vi "Car Wash.vi"() -> ()   [LabVIEW 2015]
uses:
  Controls/Car Wash Indicators.ctl
  Controls/Wash Options.ctl
  Controls/All data cluster.ctl
  Controls/#status.ctl
  Car Wash (100929B-01)/USB Template (LV 8.6)/Car Wash/Controls/#timerstatus.ctl
panel:
  in  "Wash Options":T1
  out "error out":errorcluster
  in  "error in":errorcluster
  in  "Start":bool
  out "Elapsed Time":dbl format="%0.2f"
  in  "stop":bool
  out "Wash Entry":bool
  in  "Car Position Slider":u8(slide) max=3 scale=0.0..4.0
  out "Car Wash Indicators":T2
  # "Entry Console"
  # "Car Wash Display"
  # "Car Position Simulation"
  # "Pre-Soak\nH-P Wash\nL-P Wax\nSpot Free Rinse"
  # "Underbody Wash\nBug Remover"
  # "Tire Shine\nAir Dry"
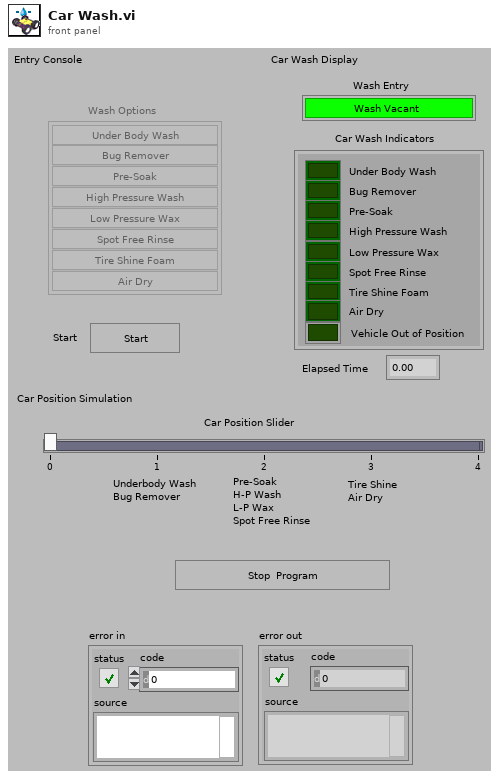
[diagram p1: front panel]
types:
  T1 = typedef "Wash Options.ctl" = cluster{"Underbody Wash":bool, "Bug Remover":bool, "Pre-Soak":bool, "High Pressure Wash":bool, "Low Pressure Wax":bool, "Spot Free Rinse":bool, "Tire Shine Foam":bool, "Air Dry":bool}
  T2 = typedef "Car Wash Indicators.ctl" = cluster{"Under Body Wash":bool, "Bug Remover":bool, "Pre-Soak":bool, "High Pressure Wash":bool, "Low Pressure Wax":bool, "Spot Free Rinse":bool, "Tire Shine Foam":bool, "Air Dry":bool, "Vehicle Out of Position":bool}
  T3 = typedef "#status.ctl" = enum16{"Error Under Range", "Skip", "Error", "Initialize", "End", "Air Dry", "Tire Shine Foam", "Spot Free Rinse", "Low Pressure Wax", "High Pressure Wash", "Pre-Soak", "Bug Remover", "Under Body Wash", "Start", "Idle", "Exit"}
  T4 = typedef "All data cluster.ctl" = cluster{"Car Wash Indicators":T2, "Wash Entry":bool, "Elapsed Time":dbl, "times":cluster{"UBW":dbl, "Bug Remover":dbl, "Pre-Soak":dbl, "HPW":dbl, "LPW":dbl, "TSF":dbl, "AD":dbl, "SFR":dbl}}
  T5 = cluster{"UBW":dbl, "Bug Remover":dbl, "Pre-Soak":dbl, "HPW":dbl, "LPW":dbl, "TSF":dbl, "AD":dbl, "SFR":dbl}
  T6 = enum8{"Enabled", "Disabled", "Disabled and Grayed Out"}
  T7 = typedef "#timerstatus.ctl" = enum16{"pause", "reset", "start"}
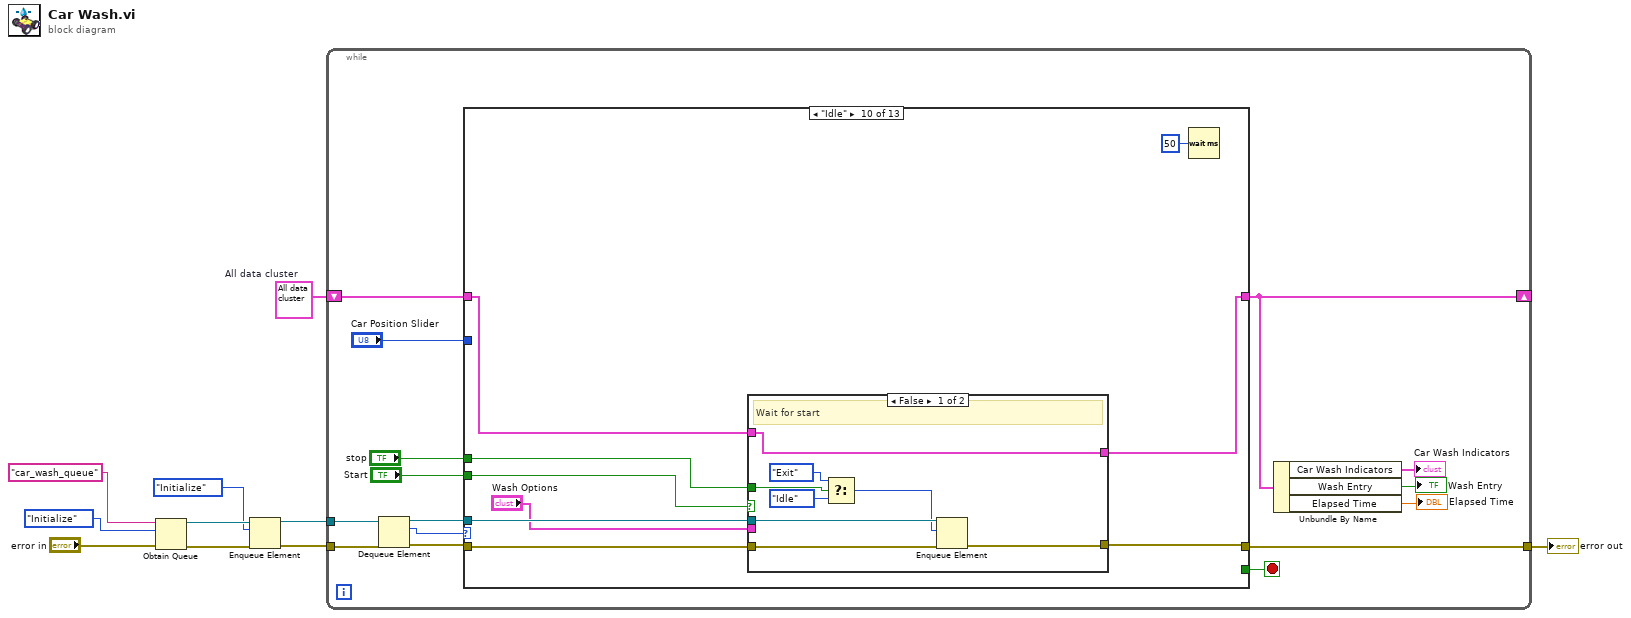
[diagram p0: block diagram]
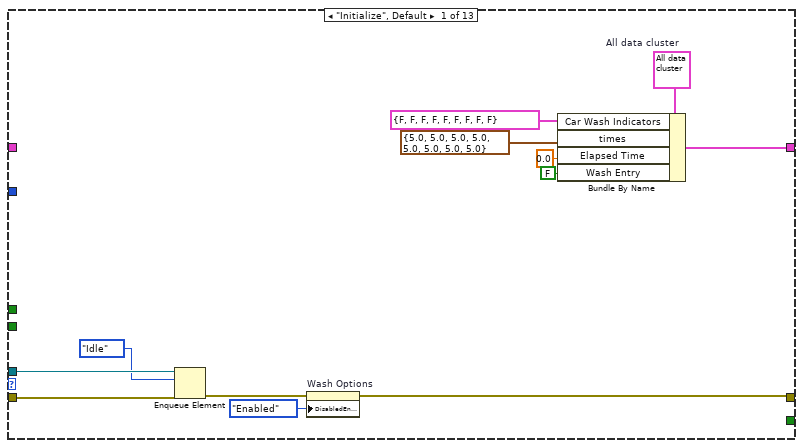
[diagram p2: hidden frame]
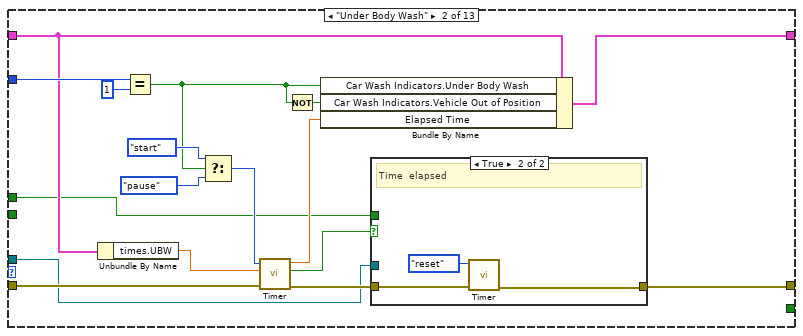
[diagram p3: hidden frame]
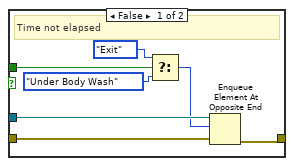
[diagram p4: hidden frame]
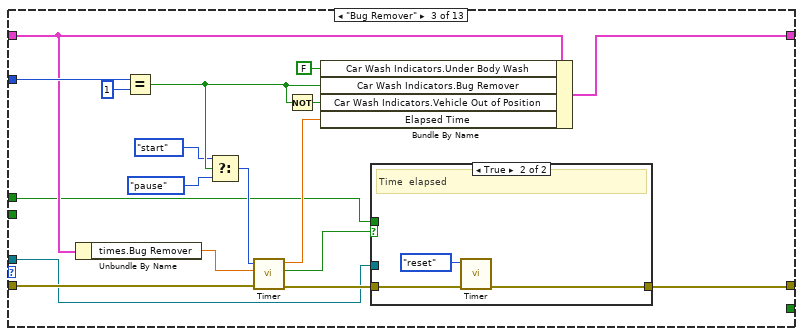
[diagram p5: hidden frame]
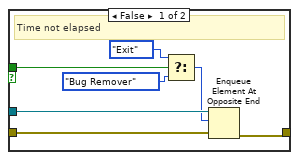
[diagram p6: hidden frame]
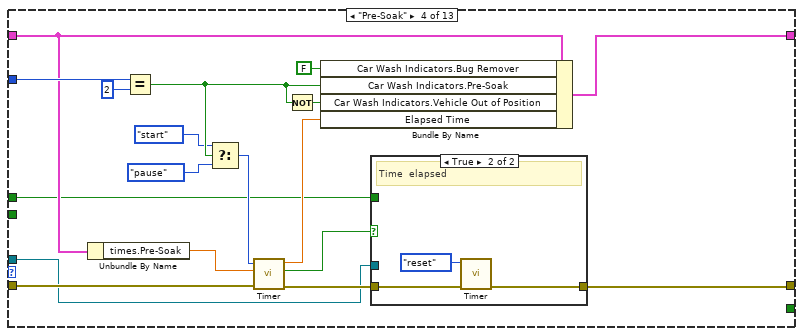
[diagram p7: hidden frame]
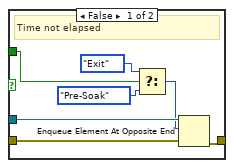
[diagram p8: hidden frame]
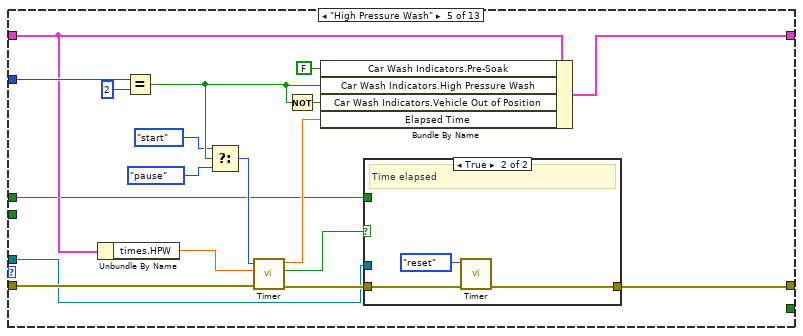
[diagram p9: hidden frame]
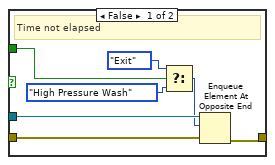
[diagram p10: hidden frame]
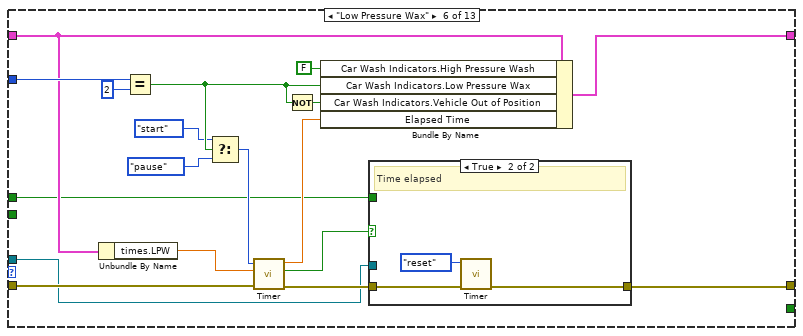
[diagram p11: hidden frame]
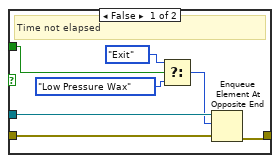
[diagram p12: hidden frame]
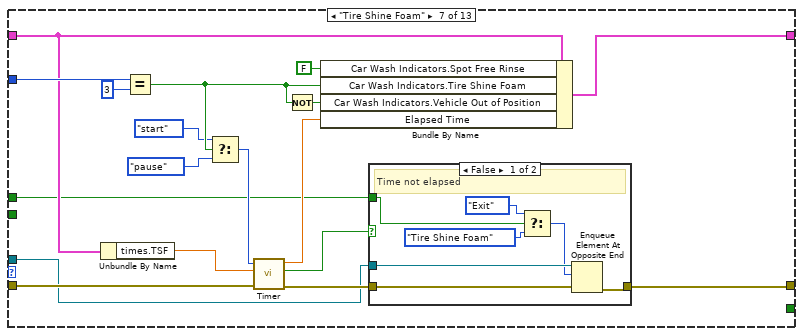
[diagram p13: hidden frame]
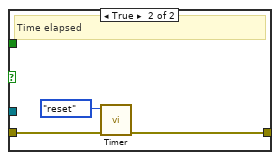
[diagram p14: hidden frame]
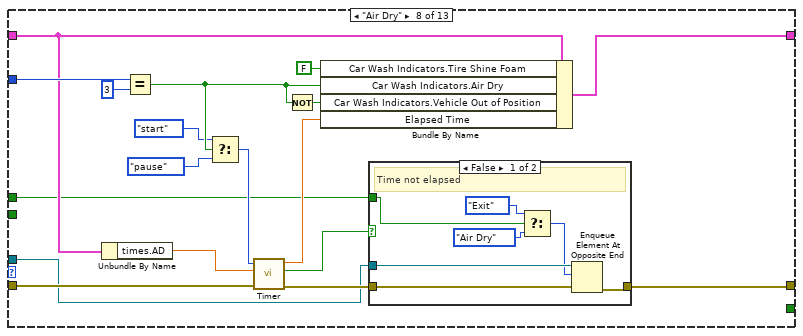
[diagram p15: hidden frame]
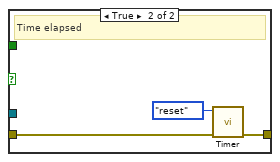
[diagram p16: hidden frame]
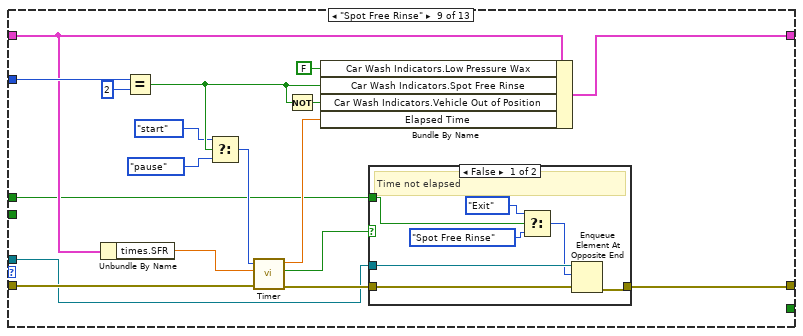
[diagram p17: hidden frame]
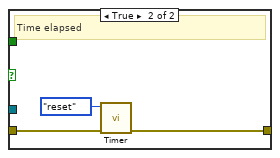
[diagram p18: hidden frame]
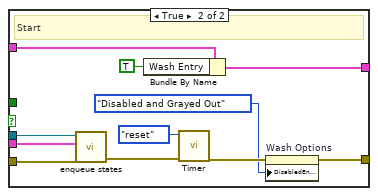
[diagram p19: hidden frame]
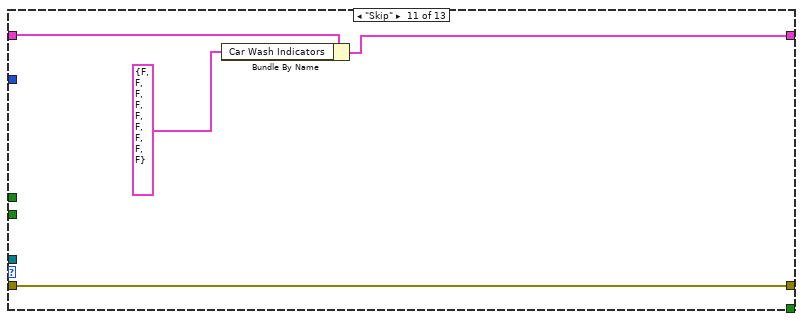
[diagram p20: hidden frame]
diagram:
  w10 = T4 {"Car Wash Indicators"={"Under Body Wash"=FALSE, "Bug Remover"=FALSE, "Pre-Soak"=FALSE, "High Pressure Wash"=FALSE, "Low Pressure Wax"=FALSE, "Spot Free Rinse"=FALSE, "Tire Shine Foam"=FALSE, "Air Dry"=FALSE, "Vehicle Out of Position"=FALSE}, "Wash Entry"=FALSE, "Elapsed Time"=0.0, "times"={"UBW"=0.0, "Bug Remover"=0.0, "Pre-Soak"=0.0, "HPW"=0.0, "LPW"=0.0, "TSF"=0.0, "AD"=0.0, "SFR"=0.0}}  # All data cluster
  n1 = Obtain Queue(name (unnamed)="car_wash_queue", element data type=#status."Initialize" ("status"), error in (no error)="error in") -> (queue out=w3:refnum<queue>, error out=w5:errorcluster)  [unwired: 2 in, 1 out]
  n2 = Enqueue Element(queue=w3, element=#status."Initialize" ("status"), error in (no error)=w5) -> (queue out=w1:refnum<queue>, error out=w4:errorcluster)  [unwired: 1 in, 1 out]
  n3 = while {
    shift-right: [w23] -> _
    shift-left: w10 -> [w24]
    tunnel: w4 -> [w18]
    tunnel: [w19] -> w9
    tunnel: w1 -> [w16]
    stop <- w25 stop-if-true
    n4 = Dequeue Element(queue=w16, error in (no error)=w18) -> (queue out=w15:refnum<queue>, element=w14:T3, error out=w17:errorcluster)  [unwired: 1 in, 1 out]
    n5 = case shown="\"Idle\"" w14 {
      tunnel: [_ _ _ _ _ _ _ _ _ _ _ _ TRUE] -> w25
      tunnel: w24 -> [_ w50 w78 w106 w134 w162 w190 w218 w246 w262 w291 w298 w317]
      tunnel: [w33 w47 w75 w103 w131 w159 w187 w215 w243 w261 w289 w295 w317] -> w23
      tunnel: w17 -> [w32 w54 w82 w110 w138 w166 w194 w222 w250 w269 w292 w304 w318]
      tunnel: [w28 w45 w73 w101 w129 w157 w185 w213 w241 w267 w292 w302 w318] -> w19
      tunnel: w15 -> [w31 w43 w71 w99 w127 w155 w183 w211 w239 w268 _ w303 _]
      tunnel: "Start" -> [_ _ _ _ _ _ _ _ _ w266 _ _ _]
      tunnel: "stop" -> [_ w38 w65 w93 w121 w149 w177 w205 w233 w265 _ _ _]
      tunnel: "Car Position Slider" -> [_ w52 w80 w108 w136 w164 w192 w220 w248 _ _ w300 _]
      frame "Initialize", Default {
        w37 = T4 {"Car Wash Indicators"={"Under Body Wash"=FALSE, "Bug Remover"=FALSE, "Pre-Soak"=FALSE, "High Pressure Wash"=FALSE, "Low Pressure Wax"=FALSE, "Spot Free Rinse"=FALSE, "Tire Shine Foam"=FALSE, "Air Dry"=FALSE, "Vehicle Out of Position"=FALSE}, "Wash Entry"=TRUE, "Elapsed Time"=0.0, "times"={"UBW"=0.0, "Bug Remover"=0.0, "Pre-Soak"=0.0, "HPW"=0.0, "LPW"=0.0, "TSF"=0.0, "AD"=0.0, "SFR"=0.0}}  # All data cluster
        n6 = Enqueue Element(queue=w31, element=#status."Idle" ("status"), error in (no error)=w32) -> (error out=w29:errorcluster)  [unwired: 1 in, 2 out]
        n7 = property on="Wash Options" class="Clust (strict)"(error in=w29, "DisabledEnum"=T6."Enabled" ("Disabled")) -> (error out=w28:errorcluster)  [unwired: 1 in, 1 out]
        n8 = Bundle By Name(cluster=w37, "Car Wash Indicators"=T2 {"Under Body Wash"=FALSE, "Bug Remover"=FALSE, "Pre-Soak"=FALSE, "High Pressure Wash"=FALSE, "Low Pressure Wax"=FALSE, "Spot Free Rinse"=FALSE, "Tire Shine Foam"=FALSE, "Air Dry"=FALSE, "Vehicle Out of Position"=FALSE}, "times"=T5 {"UBW"=5.0, "Bug Remover"=5.0, "Pre-Soak"=5.0, "HPW"=5.0, "LPW"=5.0, "TSF"=5.0, "AD"=5.0, "SFR"=5.0}, "Elapsed Time"=0.0, "Wash Entry"=FALSE) -> (w33:T4)
      }
      frame "Under Body Wash" {
        n9 = Unbundle By Name(w50) -> ("times.UBW"=w53:dbl)
        n10 = Equal?(x=w52, y=u8 1) -> (x = y?=w40:bool)
        n11 = Select(t=#timerstatus."start" ("status"), s=w40, f=#timerstatus."pause" ("status")) -> (s? t:f=w39:T7)
        n12 = call "Timer.vi"("error in"=w54, "Time limit"=w53, "status"=w39) -> ("error out"=w46:errorcluster, "elapsed"=w44:bool, "elapsed time"=w49:dbl)  [unwired: 6 in]
        n13 = Not(x=w40) -> (.not. x?=w48:bool)
        n14 = Bundle By Name(cluster=w50, "Car Wash Indicators.Under Body Wash"=w40, "Car Wash Indicators.Vehicle Out of Position"=w48, "Elapsed Time"=w49) -> (w47:T4)
        n15 = case shown="True" w44 {
          tunnel: w46 -> [w61 w64]
          tunnel: [w60 w63] -> w45
          tunnel: w43 -> [w59 _]
          tunnel: w38 -> [w56 _]
          frame False {
            # "Time not elapsed"
            n16 = Select(t=#status."Exit" ("status"), s=w56, f=#status."Under Body Wash" ("element")) -> (s? t:f=w55:T3)
            n17 = Enqueue Element At Opposite End(queue=w59, element=w55, error in (no error)=w61) -> (error out=w60:errorcluster)  [unwired: 1 in, 2 out]
          }
          frame True {
            # "Time  elapsed"
            n18 = call "Timer.vi"("error in"=w64, "status"=#timerstatus."reset") -> ("error out"=w63:errorcluster)  [unwired: 7 in, 2 out]
          }
        }
      }
      frame "Bug Remover" {
        n19 = Unbundle By Name(w78) -> ("times.Bug Remover"=w81:dbl)
        n20 = Equal?(x=w80, y=u8 1) -> (x = y?=w69:bool)
        n21 = Select(t=#timerstatus."start" ("status"), s=w69, f=#timerstatus."pause" ("status")) -> (s? t:f=w66:T7)
        n22 = call "Timer.vi"("error in"=w82, "Time limit"=w81, "status"=w66) -> ("error out"=w74:errorcluster, "elapsed"=w72:bool, "elapsed time"=w77:dbl)  [unwired: 6 in]
        n23 = Not(x=w69) -> (.not. x?=w76:bool)
        n24 = Bundle By Name(cluster=w78, "Car Wash Indicators.Under Body Wash"=FALSE, "Car Wash Indicators.Bug Remover"=w69, "Car Wash Indicators.Vehicle Out of Position"=w76, "Elapsed Time"=w77) -> (w75:T4)
        n25 = case shown="True" w72 {
          tunnel: w74 -> [w89 w92]
          tunnel: [w88 w91] -> w73
          tunnel: w71 -> [w87 _]
          tunnel: w65 -> [w83 _]
          frame False {
            # "Time not elapsed"
            n26 = Select(t=#status."Exit" ("status"), s=w83, f=#status."Bug Remover" ("element")) -> (s? t:f=w84:T3)
            n27 = Enqueue Element At Opposite End(queue=w87, element=w84, error in (no error)=w89) -> (error out=w88:errorcluster)  [unwired: 1 in, 2 out]
          }
          frame True {
            # "Time  elapsed"
            n28 = call "Timer.vi"("error in"=w92, "status"=#timerstatus."reset") -> ("error out"=w91:errorcluster)  [unwired: 7 in, 2 out]
          }
        }
      }
      frame "Pre-Soak" {
        n29 = Unbundle By Name(w106) -> ("times.Pre-Soak"=w109:dbl)
        n30 = Equal?(x=w108, y=u8 2) -> (x = y?=w97:bool)
        n31 = Select(t=#timerstatus."start" ("status"), s=w97, f=#timerstatus."pause" ("status")) -> (s? t:f=w94:T7)
        n32 = call "Timer.vi"("error in"=w110, "Time limit"=w109, "status"=w94) -> ("error out"=w102:errorcluster, "elapsed"=w100:bool, "elapsed time"=w105:dbl)  [unwired: 6 in]
        n33 = Not(x=w97) -> (.not. x?=w104:bool)
        n34 = Bundle By Name(cluster=w106, "Car Wash Indicators.Bug Remover"=FALSE ("Car Wash Indicators.Under Body Wash"), "Car Wash Indicators.Pre-Soak"=w97, "Car Wash Indicators.Vehicle Out of Position"=w104, "Elapsed Time"=w105) -> (w103:T4)
        n35 = case shown="True" w100 {
          tunnel: w102 -> [w117 w120]
          tunnel: [w116 w119] -> w101
          tunnel: w99 -> [w115 _]
          tunnel: w93 -> [w111 _]
          frame False {
            # "Time not elapsed"
            n36 = Select(t=#status."Exit" ("status"), s=w111, f=#status."Pre-Soak" ("element")) -> (s? t:f=w112:T3)
            n37 = Enqueue Element At Opposite End(queue=w115, element=w112, error in (no error)=w117) -> (error out=w116:errorcluster)  [unwired: 1 in, 2 out]
          }
          frame True {
            # "Time  elapsed"
            n38 = call "Timer.vi"("error in"=w120, "status"=#timerstatus."reset") -> ("error out"=w119:errorcluster)  [unwired: 7 in, 2 out]
          }
        }
      }
      frame "High Pressure Wash" {
        n39 = Unbundle By Name(w134) -> ("times.HPW"=w137:dbl)
        n40 = Equal?(x=w136, y=u8 2) -> (x = y?=w125:bool)
        n41 = Select(t=#timerstatus."start" ("status"), s=w125, f=#timerstatus."pause" ("status")) -> (s? t:f=w122:T7)
        n42 = call "Timer.vi"("error in"=w138, "Time limit"=w137, "status"=w122) -> ("error out"=w130:errorcluster, "elapsed"=w128:bool, "elapsed time"=w133:dbl)  [unwired: 6 in]
        n43 = Not(x=w125) -> (.not. x?=w132:bool)
        n44 = Bundle By Name(cluster=w134, "Car Wash Indicators.Pre-Soak"=FALSE ("Car Wash Indicators.Under Body Wash"), "Car Wash Indicators.High Pressure Wash"=w125, "Car Wash Indicators.Vehicle Out of Position"=w132, "Elapsed Time"=w133) -> (w131:T4)
        n45 = case shown="True" w128 {
          tunnel: w130 -> [w145 w148]
          tunnel: [w144 w147] -> w129
          tunnel: w127 -> [w143 _]
          tunnel: w121 -> [w140 _]
          frame False {
            # "Time not elapsed"
            n46 = Select(t=#status."Exit" ("status"), s=w140, f=#status."High Pressure Wash" ("element")) -> (s? t:f=w139:T3)
            n47 = Enqueue Element At Opposite End(queue=w143, element=w139, error in (no error)=w145) -> (error out=w144:errorcluster)  [unwired: 1 in, 2 out]
          }
          frame True {
            # "Time elapsed"
            n48 = call "Timer.vi"("error in"=w148, "status"=#timerstatus."reset") -> ("error out"=w147:errorcluster)  [unwired: 7 in, 2 out]
          }
        }
      }
      frame "Low Pressure Wax" {
        n49 = Unbundle By Name(w162) -> ("times.LPW"=w165:dbl)
        n50 = Equal?(x=w164, y=u8 2) -> (x = y?=w153:bool)
        n51 = Select(t=#timerstatus."start" ("status"), s=w153, f=#timerstatus."pause" ("status")) -> (s? t:f=w150:T7)
        n52 = call "Timer.vi"("error in"=w166, "Time limit"=w165, "status"=w150) -> ("error out"=w158:errorcluster, "elapsed"=w156:bool, "elapsed time"=w161:dbl)  [unwired: 6 in]
        n53 = Not(x=w153) -> (.not. x?=w160:bool)
        n54 = Bundle By Name(cluster=w162, "Car Wash Indicators.High Pressure Wash"=FALSE ("Car Wash Indicators.Under Body Wash"), "Car Wash Indicators.Low Pressure Wax"=w153, "Car Wash Indicators.Vehicle Out of Position"=w160, "Elapsed Time"=w161) -> (w159:T4)
        n55 = case shown="True" w156 {
          tunnel: w158 -> [w173 w176]
          tunnel: [w172 w175] -> w157
          tunnel: w155 -> [w171 _]
          tunnel: w149 -> [w167 _]
          frame False {
            # "Time not elapsed"
            n56 = Select(t=#status."Exit" ("status"), s=w167, f=#status."Low Pressure Wax" ("element")) -> (s? t:f=w168:T3)
            n57 = Enqueue Element At Opposite End(queue=w171, element=w168, error in (no error)=w173) -> (error out=w172:errorcluster)  [unwired: 1 in, 2 out]
          }
          frame True {
            # "Time elapsed"
            n58 = call "Timer.vi"("error in"=w176, "status"=#timerstatus."reset") -> ("error out"=w175:errorcluster)  [unwired: 7 in, 2 out]
          }
        }
      }
      frame "Tire Shine Foam" {
        n59 = Unbundle By Name(w190) -> ("times.TSF"=w193:dbl)
        n60 = Equal?(x=w192, y=u8 3) -> (x = y?=w181:bool)
        n61 = Select(t=#timerstatus."start" ("status"), s=w181, f=#timerstatus."pause" ("status")) -> (s? t:f=w178:T7)
        n62 = call "Timer.vi"("error in"=w194, "Time limit"=w193, "status"=w178) -> ("error out"=w186:errorcluster, "elapsed"=w184:bool, "elapsed time"=w189:dbl)  [unwired: 6 in]
        n63 = Not(x=w181) -> (.not. x?=w188:bool)
        n64 = Bundle By Name(cluster=w190, "Car Wash Indicators.Spot Free Rinse"=FALSE ("Car Wash Indicators.Under Body Wash"), "Car Wash Indicators.Tire Shine Foam"=w181, "Car Wash Indicators.Vehicle Out of Position"=w188, "Elapsed Time"=w189) -> (w187:T4)
        n65 = case shown="False" w184 {
          tunnel: w186 -> [w201 w204]
          tunnel: [w200 w203] -> w185
          tunnel: w183 -> [w199 _]
          tunnel: w177 -> [w195 _]
          frame False {
            # "Time not elapsed"
            n66 = Select(t=#status."Exit" ("status"), s=w195, f=#status."Tire Shine Foam" ("element")) -> (s? t:f=w196:T3)
            n67 = Enqueue Element At Opposite End(queue=w199, element=w196, error in (no error)=w201) -> (error out=w200:errorcluster)  [unwired: 1 in, 2 out]
          }
          frame True {
            # "Time elapsed"
            n68 = call "Timer.vi"("error in"=w204, "status"=#timerstatus."reset") -> ("error out"=w203:errorcluster)  [unwired: 7 in, 2 out]
          }
        }
      }
      frame "Air Dry" {
        n69 = Unbundle By Name(w218) -> ("times.AD"=w221:dbl)
        n70 = Equal?(x=w220, y=u8 3) -> (x = y?=w209:bool)
        n71 = Select(t=#timerstatus."start" ("status"), s=w209, f=#timerstatus."pause" ("status")) -> (s? t:f=w206:T7)
        n72 = call "Timer.vi"("error in"=w222, "Time limit"=w221, "status"=w206) -> ("error out"=w214:errorcluster, "elapsed"=w212:bool, "elapsed time"=w217:dbl)  [unwired: 6 in]
        n73 = Not(x=w209) -> (.not. x?=w216:bool)
        n74 = Bundle By Name(cluster=w218, "Car Wash Indicators.Tire Shine Foam"=FALSE ("Car Wash Indicators.Under Body Wash"), "Car Wash Indicators.Air Dry"=w209, "Car Wash Indicators.Vehicle Out of Position"=w216, "Elapsed Time"=w217) -> (w215:T4)
        n75 = case shown="False" w212 {
          tunnel: w214 -> [w229 w232]
          tunnel: [w228 w231] -> w213
          tunnel: w211 -> [w227 _]
          tunnel: w205 -> [w223 _]
          frame False {
            # "Time not elapsed"
            n76 = Select(t=#status."Exit" ("status"), s=w223, f=#status."Air Dry" ("element")) -> (s? t:f=w224:T3)
            n77 = Enqueue Element At Opposite End(queue=w227, element=w224, error in (no error)=w229) -> (error out=w228:errorcluster)  [unwired: 1 in, 2 out]
          }
          frame True {
            # "Time elapsed"
            n78 = call "Timer.vi"("error in"=w232, "status"=#timerstatus."reset") -> ("error out"=w231:errorcluster)  [unwired: 7 in, 2 out]
          }
        }
      }
      frame "Spot Free Rinse" {
        n79 = Unbundle By Name(w246) -> ("times.SFR"=w249:dbl)
        n80 = Equal?(x=w248, y=u8 2) -> (x = y?=w237:bool)
        n81 = Select(t=#timerstatus."start" ("status"), s=w237, f=#timerstatus."pause" ("status")) -> (s? t:f=w234:T7)
        n82 = call "Timer.vi"("error in"=w250, "Time limit"=w249, "status"=w234) -> ("error out"=w242:errorcluster, "elapsed"=w240:bool, "elapsed time"=w245:dbl)  [unwired: 6 in]
        n83 = Not(x=w237) -> (.not. x?=w244:bool)
        n84 = Bundle By Name(cluster=w246, "Car Wash Indicators.Low Pressure Wax"=FALSE ("Car Wash Indicators.Under Body Wash"), "Car Wash Indicators.Spot Free Rinse"=w237, "Car Wash Indicators.Vehicle Out of Position"=w244, "Elapsed Time"=w245) -> (w243:T4)
        n85 = case shown="False" w240 {
          tunnel: w242 -> [w257 w260]
          tunnel: [w256 w259] -> w241
          tunnel: w239 -> [w255 _]
          tunnel: w233 -> [w251 _]
          frame False {
            # "Time not elapsed"
            n86 = Select(t=#status."Exit" ("status"), s=w251, f=#status."Spot Free Rinse" ("element")) -> (s? t:f=w252:T3)
            n87 = Enqueue Element At Opposite End(queue=w255, element=w252, error in (no error)=w257) -> (error out=w256:errorcluster)  [unwired: 1 in, 2 out]
          }
          frame True {
            # "Time elapsed"
            n88 = call "Timer.vi"("error in"=w260, "status"=#timerstatus."reset") -> ("error out"=w259:errorcluster)  [unwired: 7 in, 2 out]
          }
        }
      }
      frame "Idle" {
        n89 = case shown="False" w266 {
          tunnel: w269 -> [w277 w288]
          tunnel: "Wash Options" -> [_ w287]
          tunnel: w268 -> [w275 w286]
          tunnel: [w276 w282] -> w267
          tunnel: w265 -> [w272 _]
          tunnel: w262 -> [w270 w280]
          tunnel: [w270 w279] -> w261
          frame False {
            # "Wait for start"
            n90 = Select(t=#status."Exit" ("status"), s=w272, f=#status."Idle" ("status")) -> (s? t:f=w271:T3)
            n91 = Enqueue Element(queue=w275, element=w271, error in (no error)=w277) -> (error out=w276:errorcluster)  [unwired: 1 in, 2 out]
          }
          frame True {
            # "Start"
            n92 = call "enqueue states.vi"("error in (no error)"=w288, "Wash Options"=w287, "Queue in"=w286) -> ("error out"=w284:errorcluster)  [unwired: 8 in]
            n93 = Bundle By Name(cluster=w280, "Wash Entry"=TRUE) -> (w279:T4)
            n94 = call "Timer.vi"("error in"=w284, "status"=#timerstatus."reset") -> ("error out"=w283:errorcluster)  [unwired: 7 in, 2 out]
            n95 = property on="Wash Options" class="Clust (strict)"(error in=w283, "DisabledEnum"=T6."Disabled and Grayed Out" ("Disabled")) -> (error out=w282:errorcluster)  [unwired: 1 in, 1 out]
          }
        }
        n96 = Wait (ms)(milliseconds to wait=u32 50) -> ()  [unwired: 1 out]
      }
      frame "Skip" {
        n97 = Bundle By Name(cluster=w291, "Car Wash Indicators"=T2 {"Under Body Wash"=FALSE, "Bug Remover"=FALSE, "Pre-Soak"=FALSE, "High Pressure Wash"=FALSE, "Low Pressure Wax"=FALSE, "Spot Free Rinse"=FALSE, "Tire Shine Foam"=FALSE, "Air Dry"=FALSE, "Vehicle Out of Position"=FALSE}) -> (w289:T4)
      }
      frame "End" {
        n98 = Equal?(x=w300, y=u8 4) -> (x = y?=w294:bool)
        n99 = case shown="False" w294 {
          tunnel: w304 -> [w308 w316]
          tunnel: w303 -> [w306 w315]
          tunnel: [w307 w312] -> w302
          tunnel: [TRUE FALSE] -> w293
          frame False {
            # "End of washing"
            n100 = Enqueue Element(queue=w306, element=#status."End", error in (no error)=w308) -> (error out=w307:errorcluster)  [unwired: 1 in, 2 out]
          }
          frame True {
            # "Time  elapsed"
            n101 = Enqueue Element(queue=w315, element=#status."Idle", error in (no error)=w316) -> (error out=w313:errorcluster)  [unwired: 1 in, 2 out]
            n102 = property on="Wash Options" class="Clust (strict)"(error in=w313, "DisabledEnum"=T6."Enabled" ("Disabled")) -> (error out=w312:errorcluster)  [unwired: 1 in, 1 out]
          }
        }
        n103 = Not(x=w294) -> (.not. x?=w297:bool)
        n104 = Bundle By Name(cluster=w298, "Car Wash Indicators.Air Dry"=FALSE ("Car Wash Indicators.Under Body Wash"), "Car Wash Indicators.Vehicle Out of Position"=w297, "Elapsed Time"=0.0, "Wash Entry"=w293) -> (w295:T4)
      }
      frame "Exit" {
      }
    }
    n105 = Unbundle By Name(w23) -> ("Car Wash Indicators"=→"Car Wash Indicators":T2, "Wash Entry"=→"Wash Entry":bool, "Elapsed Time"=→"Elapsed Time":dbl)
  }
  "error out" <- w9
